vi "Read Configuration Data.vi"(8 "error in (no error)":errorcluster) -> (0 "error out":errorcluster, 3 "Configuration Data":T1)   [LabVIEW 2017]
uses:
  Configuration Data.ctl
  controls/MHL Configuration.ctl
  Controller/Controller Configuration.ctl
  Boiler/Boiler Configuration.ctl
  Boiler System Globals.vi
  <vilib>/Utility/config.llb/NI_LVConfig.lvlib
  Controller/Controller.lvlib
  Boiler/Boiler.lvlib
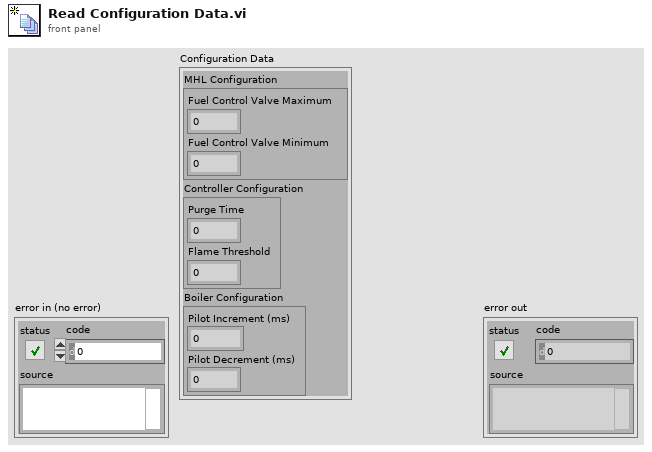
[diagram p1: front panel]
types:
  T1 = typedef "Configuration Data.ctl" = cluster{"MHL Configuration":T2, "Controller Configuration":T3, "Boiler Configuration":T4}
  T2 = typedef "MHL Configuration.ctl" = cluster{"Fuel Control Valve Maximum":dbl, "Fuel Control Valve Minimum":dbl}
  T3 = typedef "Controller.lvlib/Controller Configuration.ctl" = cluster{"Purge Time":u32, "Flame Threshold":u32}
  T4 = typedef "Boiler.lvlib/Boiler Configuration.ctl" = cluster{"Pilot Increment (ms)":u32, "Pilot Decrement (ms)":u32}
  T5 = typedef "NI_LVConfig.lvlib/Config Data RefNum.ctl" = refnum<k1>
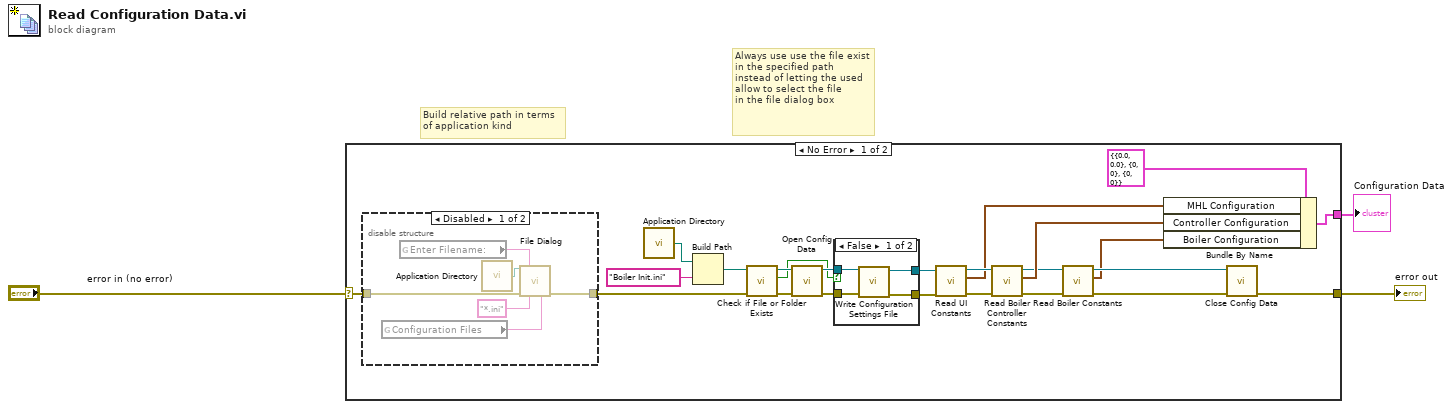
[diagram p0: block diagram]
diagram:
  # "Always use use the file exist in the specified path \ninstead of letting the used allow to select the file \nin the file dialog box"
  # "Build relative path in terms\nof application kind"
  n1 = case shown="No Error" "error in (no error)" {
    selector: "error in (no error)" -> [w27 w41]
    tunnel: [w26 w41] -> w2
    tunnel: [w9 _] -> w1
    frame No Error {
      n2 = disable-structure shown="Disabled" {
        disable-tunnel: w27 -> [w39 w40]
        disable-tunnel: [w34 w40] -> w18
        frame Disabled {
          n3 = global read "Boiler System Globals.vi" "Configuration Files"() -> (w36:string)
          n4 = global read "Boiler System Globals.vi" "Enter Filename:"() -> (w38:string)
          n5 = call <vilib>:"Application Directory.vi"() -> ("Application Directory"=w35:path)
          n6 = call "File Dialog"("start path"=w35, "prompt"=w38, "error in"=w39, "pattern (all files)"="*.ini", "pattern label"=w36) -> ("error out"=w34:errorcluster)  [unwired: 7 in, 3 out]
        }
        frame Enabled {
        }
      }
      n7 = call <vilib>:"Application Directory.vi"() -> ("Application Directory"=w25:path)
      n8 = Build Path(base path=w25, name or relative path="Boiler Init.ini") -> (appended path=w19:path)
      n9 = call <vilib>:"Check if File or Folder Exists.vi"("error in (no error)"=w18, "path"=w19) -> ("error out"=w17:errorcluster, "file or folder exists?"=w15:bool, "dup path"=w16:path)  [unwired: 7 in]
      n10 = call <vilib>:"Open Config Data.vi"("error in (no error)"=w17, "configuration file path"=w16) -> ("error out"=w24:errorcluster, "refnum"=w23:T5)  [unwired: 7 in, 1 out]
      n11 = case shown="False" w15 {
        tunnel: w24 -> [w31 w32]
        tunnel: w23 -> [w30 w33]
        tunnel: [w29 w33] -> w22
        tunnel: [w28 w32] -> w21
        frame False {
          n12 = call "Write Configuration Settings File.vi"("error in (no error)"=w31, "refnum"=w30) -> ("error out"=w28:errorcluster, "refnum out"=w29:T5)  [unwired: 8 in]
        }
        frame True {
        }
      }
      n13 = call "Read UI Constants.vi"("error in (no error)"=w21, "CFG File Refnum in"=w22) -> ("error out"=w14:errorcluster, "MHL Configuration"=w11:T2, "refnum out"=w13:T5)  [unwired: 7 in]
      n14 = call "Read Boiler Controller Constants.vi"("error in"=w14, "CFG File Refnum in"=w13) -> ("error out"=w8:errorcluster, "Controller Configuration"=w10:T3, "CFG File Refnum out"=w6:T5)  [unwired: 7 in]
      n15 = call "Read Boiler Constants.vi"("error in"=w8, "CFG File Refnum in"=w6) -> ("error out"=w7:errorcluster, "Boiler Configuration"=w4:T4, "CFG File Refnum out"=w5:T5)  [unwired: 7 in]
      n16 = Bundle By Name(cluster=T1 {"MHL Configuration"={"Fuel Control Valve Maximum"=0.0, "Fuel Control Valve Minimum"=0.0}, "Controller Configuration"={"Purge Time"=0, "Flame Threshold"=0}, "Boiler Configuration"={"Pilot Increment (ms)"=0, "Pilot Decrement (ms)"=0}} ("Configuration Data"), "MHL Configuration"=w11, "Controller Configuration"=w10, "Boiler Configuration"=w4) -> (w9:T1)
      n17 = call <vilib>:"Close Config Data.vi"("error in (no error)"=w7, "refnum"=w5) -> ("error out"=w26:errorcluster)  [unwired: 8 in, 1 out]
    }
    frame Error {
    }
  }
  "error out" <- w2
  "Configuration Data" <- w1
